vi "get_temporary_file_folder_path.vi"(8 "error in (no error)":errorcluster, 11 "Image in":refnum<class "Image.lvclass">) -> (0 "error out":errorcluster, 2 "temp file folder":path, 3 "Image out":refnum<class "Image.lvclass">)   [LabVIEW 2010, in "Image.lvclass"]
uses:
  Image.lvclass
  class_data.vi
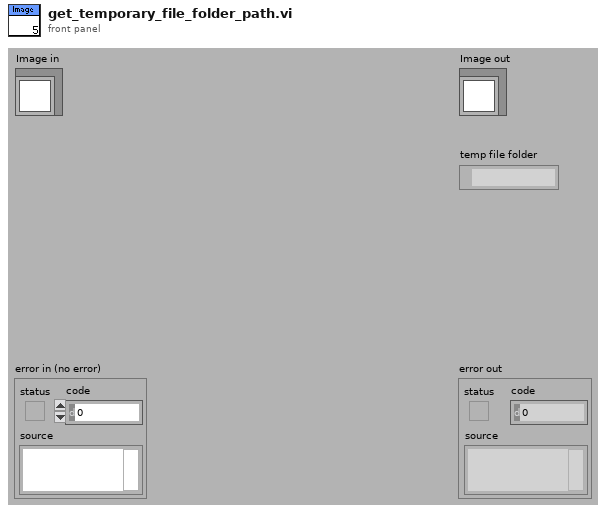
[diagram p1: front panel]
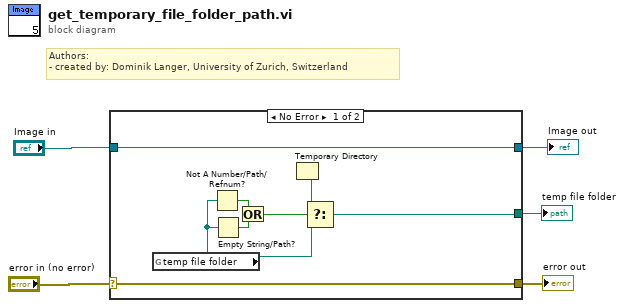
[diagram p0: block diagram]
diagram:
  # "Authors: \n- created by: Dominik Langer, University of Zurich, Switzerland"
  n1 = case shown="No Error" "error in (no error)" {
    selector: "error in (no error)" -> [w12 w15]
    tunnel: [w12 w15] -> w4
    tunnel: [w13 w14] -> w2
    tunnel: "Image in" -> [w13 w14]
    tunnel: [w6 _] -> w1
    frame No Error {
      n2 = global read "class_data.vi" "temp file folder"() -> (w8:path)
      n3 = Not A Number/Path/Refnum?(number/path/refnum=w8) -> (NaN/Path/Refnum?=w10:bool)
      n4 = Empty String/Path?(string/path=w8) -> (empty?=w11:bool)
      n5 = Or(x=w10, y=w11) -> (x .or. y?=w9:bool)
      n6 = Temporary Directory() -> (w7:path)
      n7 = Select(t=w7, s=w9, f=w8) -> (s? t:f=w6:path)
    }
    frame Error {
    }
  }
  "error out" <- w4
  "Image out" <- w2
  "temp file folder" <- w1
